vi "Periodic Tasks.vi"(8 "error in":errorcluster) -> ()   [LabVIEW 2016]
doc: "This VI runs in parallel to other tasks. It can contain as many user-defined periodic loops as you need. These can carry out PID or other sorts of timed response."
uses:
  <vilib>/Rock Robotics/WPI/Utilities/WPI_GetSetVariantRefNum.vi
  <vilib>/Rock Robotics/WPI/Ultrasonic/WPI_SonarMB1010AnalogRefNum Registry Get.vi
  <vilib>/Rock Robotics/Network Tables/NT Write Numeric Array.vi
  Robot Global Data.vi
  <vilib>/Rock Robotics/WPI/Ultrasonic/WPI_SonarMB1010AnalogGetRange.vi
  <vilib>/Rock Robotics/Network Tables/NT Write Number.vi
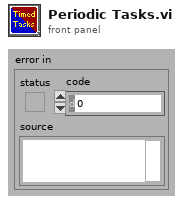
[diagram p1: front panel]
types:
  T1 = typedef "WPI_JoystickDevRef.ctl" = cluster{"Device":T2}
  T2 = typedef "WPI_JoystickDeviceEnum.ctl" = enum16{"USB 0", "USB 1", "USB 2", "USB 3", "USB 4", "USB 5"}
  T3 = typedef "WPI_SonarMB1010AnalogDeviceRef.ctl" = cluster{"AIDeviceRef":T4, "Scaling factor (V/in)":dbl, "Average Bits":u8}
  T4 = typedef "WPI_AnalogChannelDevRef.ctl" = cluster{"DevStatus":errorcluster, "Analog Channel":T5}
  T5 = typedef "FPGA_AIChannel.ctl" = enum8{"AI 0", "AI 1", "AI 2", "AI 3", "AI MXP 0", "AI MXP 1", "AI MXP 2", "AI MXP 3", "Invalid"}
  T6 = cluster{"JoystickDevRef":T1, "SonarMB1010AnalogDevRef":T3}
  T7 = cluster{"Yaw":dbl, "Roll":dbl, "Pitch":dbl, "Heading":dbl, "Fused Heading":dbl}
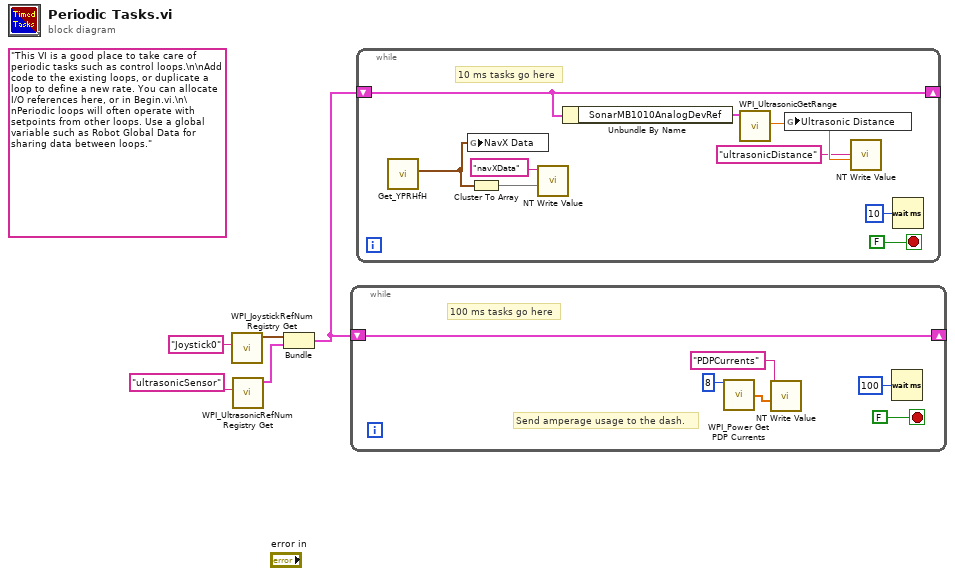
[diagram p0: block diagram]
diagram:
  (unwired) "This VI is a good place to take care of periodic tasks such as control loops.\n\nAdd code to the existing loops, or duplicate a loop to define a new rate. You can allocate I/O references here, or in Begin.vi.\n\nPeriodic loops will often operate with setpoints from other loops. Use a global variable such as Robot Global Data for sharing data between loops."
  n1 = call <vilib>:"WPI_JoystickRefNum Registry Get.vi"("refnum name"="Joystick0") -> ("JoystickDevRef"=w4:T1)  [unwired: 1 in, 9 out]
  n2 = call-poly <vilib>:"WPI_UltrasonicRefNum Registry Get.vi"("refnum name"="ultrasonicSensor") -> ("SonarMB1010AnalogDevRef"=w1:T3)  [unwired: 9 in, 1 out]
  n3 = Bundle("JoystickDevRef"=w4, "SonarMB1010AnalogDevRef"=w1) -> (w3:T6)  [unwired: 1 out]
  n4 = while {
    shift-right: [w6] -> _
    shift-left: w3 -> [w6]
    stop <- FALSE stop-if-true
    # "Send amperage usage to the dash."
    # "100 ms tasks go here"
    n5 = call <vilib>:"WPI_Power Get PDP Currents.vi"("Power Distribution Panel (0)"=u8 8) -> ("all currents (A)"=w9:dbl[])  [unwired: 12 in, 2 out]
    n6 = call-poly <vilib>:"NT Write Value.vi"("Numeric Array"=w9, "Name"="PDPCurrents") -> ()  [unwired: 9 in, 1 out]
    n7 = Wait (ms)(milliseconds to wait=u32 100) -> ()  [unwired: 1 out]
  }
  n8 = while {
    shift-right: [w15] -> _
    shift-left: w3 -> [w15]
    stop <- FALSE stop-if-true
    # "10 ms tasks go here"
    n9 = call <vilib>:"Get_YPRHfH.vi"() -> ("YRPHfH"=w12:T7)  [unwired: 11 in]
    n10 = global write "Robot Global Data.vi" "NavX Data"(w12) -> ()
    n11 = Cluster To Array(cluster=w12) -> (array=w13:dbl[])
    n12 = call-poly <vilib>:"NT Write Value.vi"("Numeric Array"=w13, "Name"="navXData") -> ()  [unwired: 9 in, 1 out]
    n13 = Unbundle By Name(w15) -> ("SonarMB1010AnalogDevRef"=w18:T3)
    n14 = call-poly <vilib>:"WPI_UltrasonicGetRange.vi"("SonarMB1010AnalogDevRef"=w18) -> ("Distance"=w17:dbl)  [unwired: 8 in, 2 out]
    n15 = global write "Robot Global Data.vi" "Ultrasonic Distance"(w17) -> ()
    n16 = call-poly <vilib>:"NT Write Value.vi"("Numeric"=w17, "Name"="ultrasonicDistance") -> ()  [unwired: 9 in, 1 out]
    n17 = Wait (ms)(milliseconds to wait=u32 10) -> ()  [unwired: 1 out]
  }
